vi "Test Parsing Simple Example CaseStructure 1.vi"() -> ()   [LabVIEW 2014]
panel:
  out "CaseStructure calls":string[](array[string])
  out "error out 2":errorcluster
  out "element translation order":string[](array[string])
  in  "vi path":path=path "C:/Users/lubo/Documents/LabView/LabVIEW-Universal-Transcriptor/Test/Examples For Parsing/Example CaseStructure 2.vi"
  # "Everything is for noqw stored inside string list, so it means that all callected WhileLoops, SubVIs transcripted C code are store separately and after parsing there is generating them to output, but they are interleaved instead recursive nested, so this is what needs to repair next."
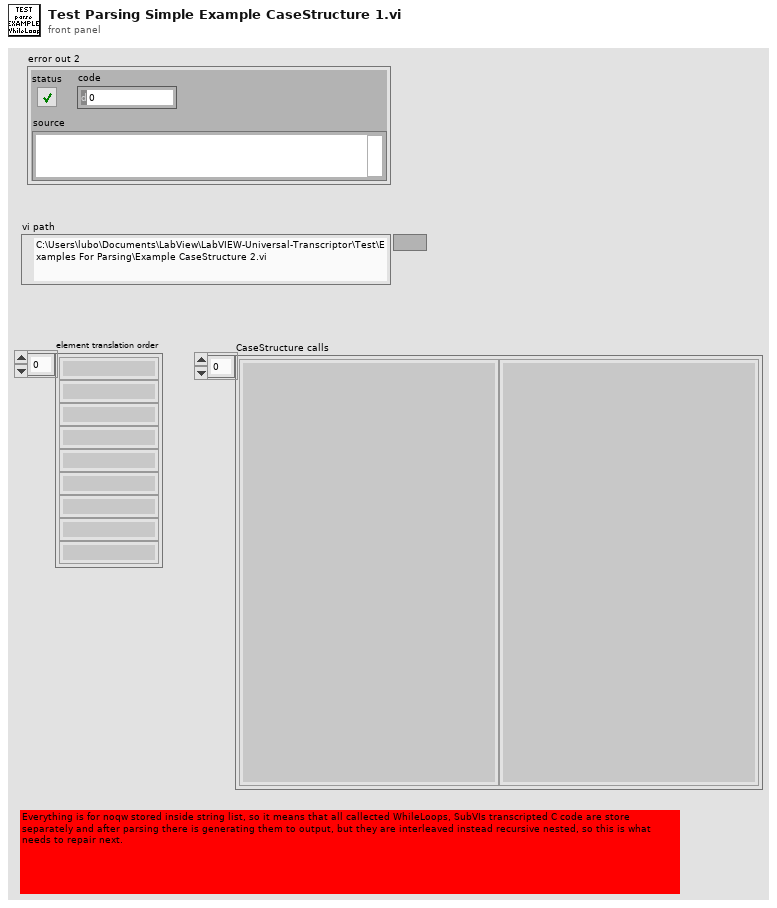
[diagram p1: front panel]
types:
  T1 = cluster{"terminals datatypes":string[][], "terminal\nconnected?":bool[], "terminal captions":string[], "term. count":i32, "terminal\nIsSource?":bool[], "SubVI name":string, "connected\nwires refs.":refnum<vi>[], "coerced\ndot?":bool[]}
  T2 = cluster{"output vars declaration":string, "output assignemnts":string, "complete code":string, "inside declarations":string}
  T3 = cluster{"terminals datatypes":string[][], "terminal\nconnected?":bool[], "terminal captions":string[], "term. count":i32, "terminal\nIsSource?":bool[], "SubVI name":string, "connected\nwires refs.":refnum<vi>[], "coerced dot?":bool[]}
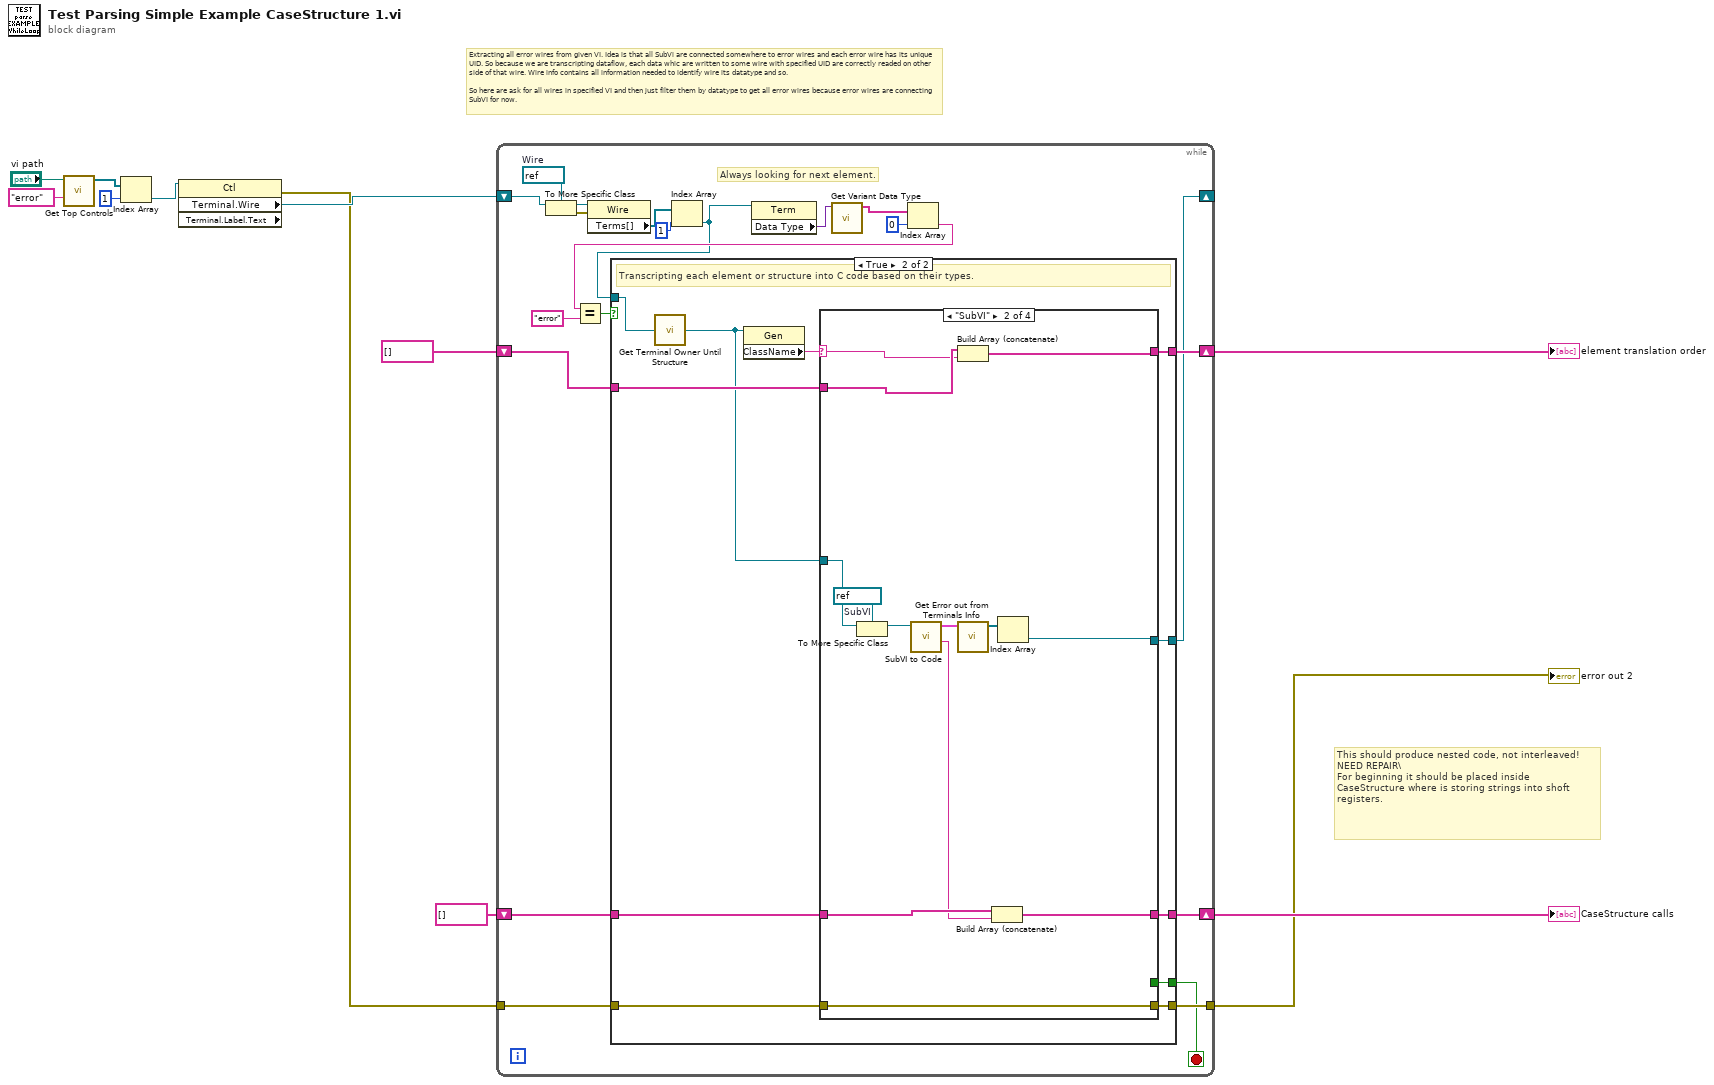
[diagram p0: block diagram]
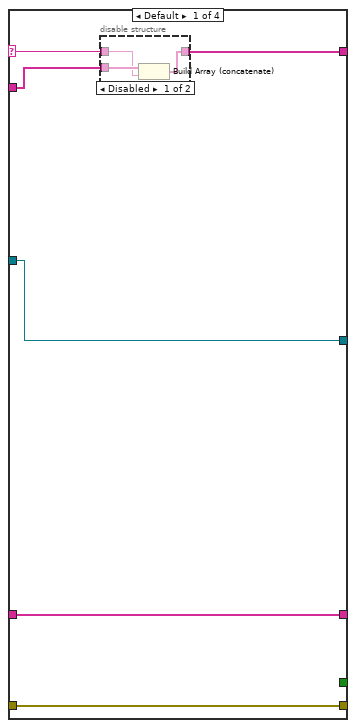
[diagram p3: hidden frame]
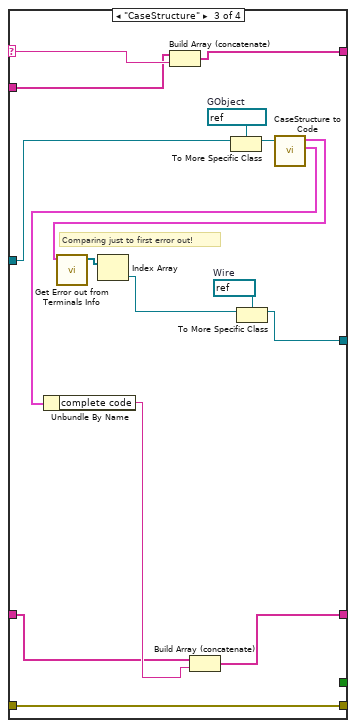
[diagram p5: hidden frame]
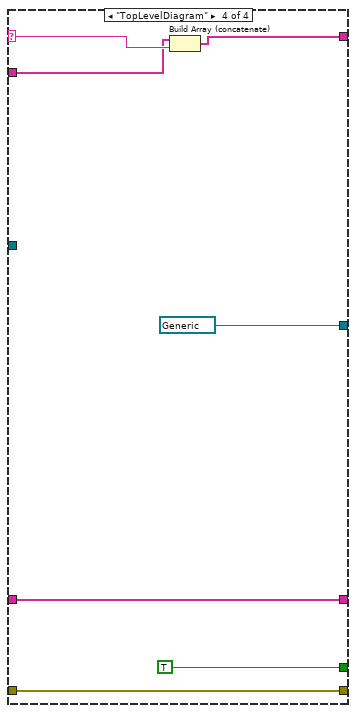
[diagram p6: hidden frame]
diagram:
  # "This should produce nested code, not interleaved!\nNEED REPAIR\\\nFor beginning it should be placed inside CaseStructure where is storing strings into shoft registers."
  # "Extracting all error wires from given VI. Idea is that all SubVi are connected somewhere to error wires and each error wire has its unique UID. So because we are transcripting dataflow, each data whic are written to some wire with specified UID are correctly readed on other side of that wire. Wire info contains all information needed to identify wire its datatype and so.\n\nSo here are ask for all wires in specified VI and then just filter them by datatype to get all error wires because error wires are connecting SubVI for now."
  n1 = call "Get Top Controls.vi"("DataType"="error", "vi path"="vi path") -> ("Controls Referencies Array"=w9:refnum<vi>[])  [unwired: 8 in, 1 out]
  n2 = Index Array(array=w9, index=1) -> (element=w8:refnum<vi>)
  n3 = property class="Ctl" props=["Terminal", "Wire", "Terminal", "Label", "Text"](reference=w8) -> (error out=w5:errorcluster, "Terminal.Wire"=w7:refnum<vi>)  [unwired: 1 in, 2 out]
  n4 = while {
    shift-right: [w22] -> w2
    shift-left: string[] [] -> [w21]
    shift-right: [w19] -> w3
    shift-left: string[] [] -> [w18]
    tunnel: [w16] -> w1
    tunnel: w5 -> [w15]
    shift-right: [w14] -> _
    shift-left: w7 -> [w17]
    stop <- w13 stop-if-true
    w33 = refnum<vi> refnum  # Wire
    # "Always looking for next element."
    n5 = To More Specific Class(target class=w33, reference=w17) -> (specific class reference=w24:refnum<vi>, error out=w32:errorcluster)  [unwired: 1 in]
    n6 = property class="Wire"(reference=w24, error in=w32) -> ("Terms[]"=w31:refnum<vi>[])  [unwired: 2 out]
    n7 = Index Array(array=w31, index=1) -> (element=w20:refnum<vi>)
    n8 = property class="Term"(reference=w20) -> ("Data Type"=w30:variant)  [unwired: 1 in, 2 out]
    n9 = call "Get Variant Data Type.vi"("variant"=w30) -> ("Data Type"=w29:string[])  [unwired: 10 in]
    n10 = Index Array(array=w29, index=0) -> (element=w27:string)
    n11 = Equal?(x=w27, y="error") -> (x = y?=w23:bool)
    n12 = case shown="True" w23 {
      tunnel: [w37 w43] -> w22
      tunnel: w21 -> [w37 w47]
      tunnel: w20 -> [w34 w48]
      tunnel: [w36 w41] -> w19
      tunnel: w18 -> [w36 w39]
      tunnel: [w35 w45] -> w16
      tunnel: w15 -> [w35 w46]
      tunnel: [w34 w42] -> w14
      tunnel: [_ w44] -> w13
      frame False {
      }
      frame True {
        # "Transcripting each element or structure into C code based on their types."
        n13 = call "Get Terminal Owner Until Structure.vi"("Term Refnum"=w48) -> ("structure ref"=w38:refnum<vi>)
        n14 = property class="Gen"(reference=w38) -> ("ClassName"=w40:string)  [unwired: 1 in, 2 out]
        n15 = case shown="\"SubVI\"" w40 {
          selector: w40 -> [w52 w66 w85 w92]
          tunnel: w38 -> [w49 w70 w76 _]
          tunnel: [w54 w68 w77 w94] -> w43
          tunnel: w47 -> [w54 w69 w75 w94]
          tunnel: [w51 w65 w86 w93] -> w41
          tunnel: w39 -> [w53 w67 w84 w91]
          tunnel: [w50 w64 w83 w90] -> w45
          tunnel: w46 -> [w50 w64 w83 w90]
          tunnel: [w49 w59 w72 refnum<vi> refnum ("Owner")] -> w42
          tunnel: [_ _ _ TRUE] -> w44
          frame Default {
            n16 = disable-structure shown="Disabled" {
              disable-tunnel: w53 -> [w57 w58]
              disable-tunnel: w52 -> [w56 _]
              disable-tunnel: [w55 w58] -> w51
              frame Disabled {
                n17 = Build Array (concatenate)(w57, w56) -> (w55:string[])
              }
              frame Enabled {
              }
            }
          }
          frame "SubVI" {
            w71 = refnum<vi> refnum  # SubVI
            n18 = To More Specific Class(target class=w71, reference=w70) -> (specific class reference=w63:refnum<vi>)  [unwired: 1 in, 1 out]
            n19 = call "SubVI to Code.vi"("reference"=w63) -> ("SubVI C call"=w62:string, "SubVI terminals info"=w60:T1)  [unwired: 8 in, 1 out]
            n20 = Build Array (concatenate)(w67, w66) -> (w65:string[])
            n21 = call "Get Error out from Terminals Info.vi"("terminals info"=w60) -> ("error out wires"=w61:refnum<vi>[])  [unwired: 9 in, 1 out]
            n22 = Build Array (concatenate)(w69, w62) -> (w68:string[])
            n23 = Index Array(array=w61) -> (element=w59:refnum<vi>)  [unwired: 1 in]
          }
          frame "CaseStructure" {
            w74 = refnum<vi> refnum  # Wire
            w87 = refnum<vi> refnum  # GObject
            # "Comparing just to first error out!"
            n24 = Build Array (concatenate)(w84, w85) -> (w86:string[])
            n25 = To More Specific Class(target class=w87, reference=w76) -> (specific class reference=w80:refnum<vi>)  [unwired: 1 in, 1 out]
            n26 = call "CaseStructure to Code.vi"("case struct ref."=w80) -> ("CaseStructure code chunks"=w81:T2, "terminals info"=w79:T3)  [unwired: 8 in, 1 out]
            n27 = Unbundle By Name(w81) -> ("complete code"=w82:string)
            n28 = call "Get Error out from Terminals Info.vi"("terminals info"=w79) -> ("error out wires"=w78:refnum<vi>[])  [unwired: 9 in, 1 out]
            n29 = Index Array(array=w78) -> (element=w73:refnum<vi>)  [unwired: 1 in]
            n30 = Build Array (concatenate)(w75, w82) -> (w77:string[])
            n31 = To More Specific Class(target class=w74, reference=w73) -> (specific class reference=w72:refnum<vi>)  [unwired: 1 in, 1 out]
          }
          frame "TopLevelDiagram" {
            n32 = Build Array (concatenate)(w91, w92) -> (w93:string[])
          }
        }
      }
    }
  }
  "element translation order" <- w3
  "error out 2" <- w1
  "CaseStructure calls" <- w2
